vi "Insert Key Value Pair (Nested Numeric Array).vi"(7 "key":string[](array[string]), 8 "error in (no error)":errorcluster, 10 "JSON Data in":dbl[](array[numeric]), 11 "JSON Object in":refnum<class "JSON Object.lvclass">) -> (0 "error out":errorcluster, 1 "replaced":bool, 3 "JSON Object Out":refnum<class "JSON Object.lvclass">)   [LabVIEW 2015, in "LVJSON.lvlib" / "JSON Object.lvclass"]
uses:
  JSON Object.lvclass
  JSON Array/New JSON Array (Numeric).vi
  JSON Helper/JSON Helper.lvclass
  JSON Array/JSON Array.lvclass
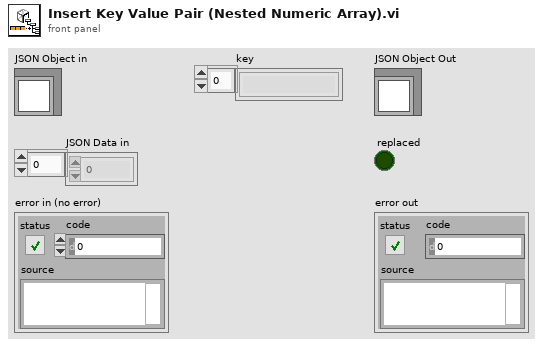
[diagram p1: front panel]
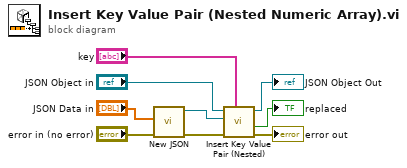
[diagram p0: block diagram]
diagram:
  n1 = call-poly "New JSON.vi"("error in (no error)"="error in (no error)", "Numeric Array"="JSON Data in") -> ("error out"=w8:errorcluster, "JSON Array out"=w9:refnum<class "JSON Array.lvclass">)  [unwired: 8 in]
  n2 = call "Insert Key Value Pair (Nested).vi"("key"="key", "error in (no error)"=w8, "JSON Data in"=w9, "JSON Object in"="JSON Object in") -> ("error out"=→"error out":errorcluster, "replaced"=→"replaced":bool, "JSON Object Out"=→"JSON Object Out":refnum<class "JSON Object.lvclass">)  [unwired: 5 in]
